vi "gfitsio-get-num-hdus.vi"(8 "error in (no error)":errorcluster, 11 "gfits refnum":T1) -> (0 "error out":errorcluster, 2 "number of hdus":i32, 3 "dup gfits refnum":T1)   [LabVIEW 2014, in "gfitsio.lvlib"]
doc: "Return the total number of HDUs in the FITS file. This returns the number of completely defined HDUs in the file. If a new HDU has just been added to the FITS file, then that HDU will only be counted if it has been closed, or if data has been written to the HDU. The current HDU remains unchanged by this VI."
uses:
  gfitsio.lvlib
  gfitsio-refnum.ctl
  gfitsio.dll
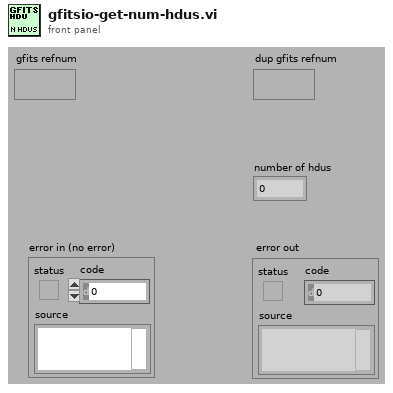
[diagram p1: front panel]
types:
  T1 = typedef "gfitsio.lvlib/gfitsio-refnum.ctl" = refnum<k1>
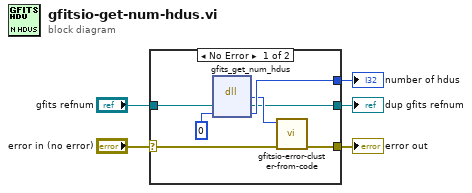
[diagram p0: block diagram]
diagram:
  n1 = case shown="No Error" "error in (no error)" {
    selector: "error in (no error)" -> [w10 w14]
    tunnel: [w9 w14] -> w5
    tunnel: "gfits refnum" -> [w7 w13]
    tunnel: [w8 w13] -> w3
    tunnel: [w12 _] -> w1
    frame No Error {
      n2 = dll-call lib="D:/optics_and_proj_related_stuff/labview_codes/gfitsio/gfitsio.dll" fn="gfits_get_num_hdus"("gfits refnum"=w7, "numhdus"=0) -> (w11:i32, "gfits refnum"=w8:T1, "numhdus"=w12:i32)  [unwired: 3 in, 2 out]
      n3 = call "gfitsio-error-cluster-from-code.vi"("error in (no error)"=w10, "error code"=w11) -> ("error out"=w9:errorcluster)  [unwired: 9 out]
    }
    frame Error {
    }
  }
  "error out" <- w5
  "dup gfits refnum" <- w3
  "number of hdus" <- w1
